vi "Transfer Command Handler.vi"(11 "Buttons":bool[](array[boolean])) -> ()   [LabVIEW 2019]
uses:
  35ffef5c-5007-404d-b716-8f1546b73e01.vi
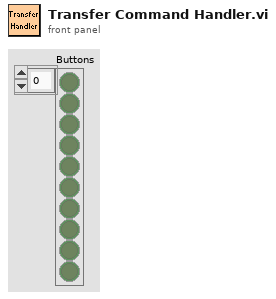
[diagram p1: front panel]
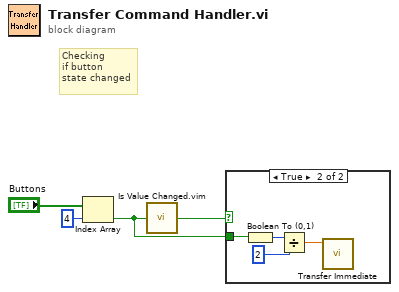
[diagram p0: block diagram]
diagram:
  # "Checking\nif button\nstate changed"
  n1 = Index Array(array="Buttons", index=4) -> (element=w1:bool)
  n2 = call "Is Value Changed.vim"("value"=w1) -> ("changed or first call?"=w2:bool)
  n3 = case shown="True" w2 {
    tunnel: w1 -> [_ w7]
    frame False {
    }
    frame True {
      n4 = Boolean To (0,1)(Boolean=w7) -> (0, 1=w8:i16)
      n5 = Divide(x=w8, y=i16 2) -> (x/y=w5:dbl)
      n6 = call "Transfer Immediate.vi"("Setpoint"=w5) -> ()  [unwired: 10 in, 1 out]
    }
  }
